vi "Add Subordinate.vi"(8 "error in":errorcluster, 10 "Subordinate":T1, 11 "Base Software in":refnum<class "Base Software.lvclass">) -> (0 "error out":errorcluster, 3 "Base Software out":refnum<class "Base Software.lvclass">)   [LabVIEW 2019, in "Base Software.lvlib" / "Main.lvlib" / "Base Software.lvclass"]
uses:
  Project/Base Software.lvclass
  Custom Controls/Subordinate.ctl
  builds/Engine/Actor Framework.lvlibp/1abvi3w/vi.lib/ActorFramework/Message Enqueuer/Message Enqueuer.lvclass
  Custom Controls/Panel_Positions.ctl
  Project/Base Software.lvclass/Base Software.ctl
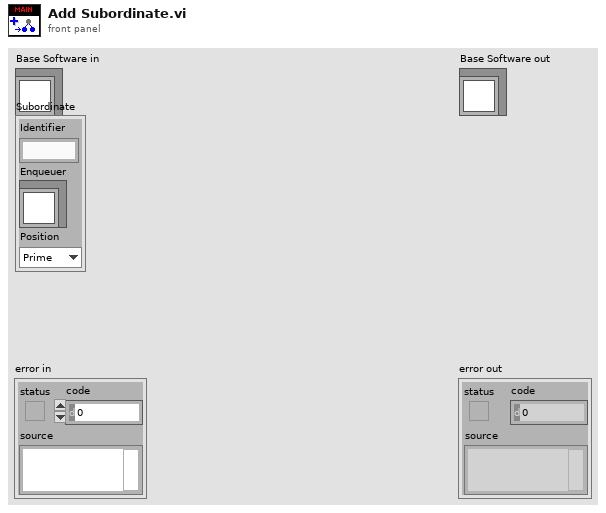
[diagram p1: front panel]
types:
  T1 = typedef "Base Software.lvlib/Main.lvlib/Base Software.lvclass/Subordinate.ctl" = cluster{"Identifier":string, "Enqueuer":refnum<class "Message Enqueuer.lvclass">, "Position":T2}
  T2 = typedef "Base Software.lvlib/Main.lvlib/Base Software.lvclass/Panel_Positions.ctl" = enum16{"Prime", "Right", "Bottom", "Left", "Mission"}
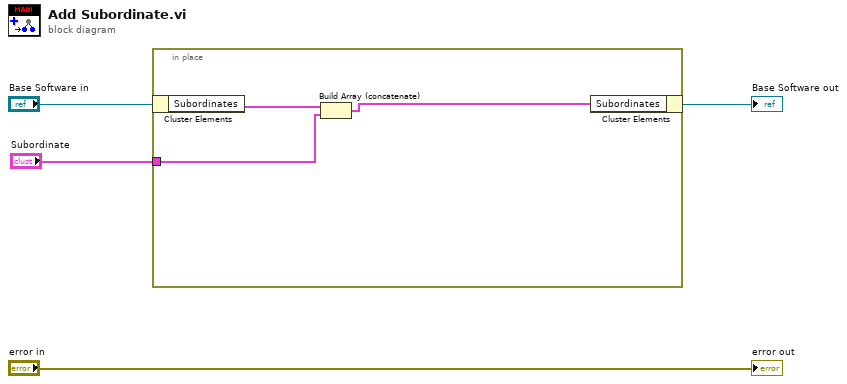
[diagram p0: block diagram]
diagram:
  n1 = in-place {
    in-place-border: "Subordinate" -> [w5]
    n2 = in-place-cluster #1("Base Software in") -> ("Subordinates"=w7:T1[])
    n3 = Build Array (concatenate)(w7, w5) -> (w6:T1[])
    n4 = in-place-cluster #1("Subordinates"=w6) -> (→"Base Software out":refnum<class "Base Software.lvclass">)
  }
  "error out" <- "error in"
